vi "Fetch Multiple Records.vi"(0 "device session in":refnum<class "Device Session.lvclass">, 1 "starting record":u64, 2 "number of records":u64=1, 5 "fetch relative to":T1=enum."First Pretrigger Sample", 7 "number of samples":u64=1000, 9 "timeout (ms)":i32=1000, 11 "error in":errorcluster, 12 "fetch offset":i64, 13 "channel":u8=1) -> (4 "device session out":refnum<class "Device Session.lvclass">, 6 "data":dbl[][](array[numeric]), 8 "relativeX (samples)":dbl[](array[numeric]), 14 "requested records info":T2[](array[typedef]), 15 "error out":errorcluster)   [LabVIEW 2021, in "Device Session.lvclass"]
doc: "Fetches data from multiple records in an acquisition. No data is returned if this VI times out. You must run the <B>Initiate</B> VI before running this VI.\n\n<B>Input Parameters</B>\n\n<B>device session in</B> is a reference to the Device Session object, which contains a session to each instrument design library used in this sample project. This parameter is obtained from the 'Open Session' VI.\n\n<B>number of records</B> specifies the number of records to fetch samples from. The default value is 1.\n\n<B>starting record</B> specifies the record to retrieve. Index of the record numbers starts at 0.\n\n<B>fetch relative to</B> specifies the relative location within the acquired record from where the VI begins to fetch data.\n\n'First Sample': the fetch starts at the first sample acquired by the device. If the device wraps data in its memory buffer, the first sample is no longer available. In this case, the VI returns an error if 'fetch offset' specifies a location that is within the overwritten portion of the memory buffer.\n'Reference Trigger Sample': the fetch starts relative to the Reference Trigger.\n'First Pretrigger Sample': the fetch starts relative to the first pretrigger sample acquired. If you do not configure a Reference Trigger, 'First Pretrigger Sample' behaves the same as 'First Sample' because there are no pretrigger samples.\n'Most Recent Sample': the fetch starts relative to the most recently acquired sample. The value of 'fetch offset' must be negative. This VI doesn't support this option. Consider using the 'Fetch Single Record' VI instead.\n'Current Read Position': the fetch starts after the last fetched sample. This VI doesn't support this option. Consider using the 'Fetch Single Record' VI instead.\n\n<B>number of samples</B> specifies the number of samples to fetch. The default value is 1000.\n\n<B>timeout (ms)</B> specifies the time, in milliseconds, allotted for the Fetch Multiple Records VI to complete execution of each record before returning a timeout error. A value of -1 specifies that the VI waits until all data is available. A value of 0 is not supported. The default value is 10,000. You cannot abort a pending fetch using the Abort VI or Close VI.\n\n<B>fetch offset</B> specifies the offset relative to the position, which is specified by the 'fetch relative to' parameter, from which to start fetching data. Offset can be a positive or negative value. The default value is 0.\n\n<B>error in</B> describes error conditions that occur before this node runs. This input provides standard 'error in' functionality.\n\n<B>Output Parameters</B>\n\n<B>device session out</B> passes a reference to the session to the next VI.\n\n<B>data</B> returns the acquired records. Each waveform corresponds to a record. If the fetch contains multiple channels, all waveforms for a record are returned before proceeding to the next record. For example, a two-channel, two-record acquisition returns four waveforms:\narray index 0 = Channel0 Record0\narray index 1 = Channel1 Record0\narray index 2 = Channel0 Record1\narray index 3 = Channel1 Record1\n\n<B>relativeX (samples)</B> returns the relative positions from the trigger to the first sample in the acquired data.\n\n<B>requested records info</B> returns additional information about each record returned by 'data'. There is one element in the 'requested records info' array for each record.\n\n<B>requested records info.number of samples</B> returns the number of samples in the record.\n\n<B>requested records info.starting sample number</B> returns the sample number of the first sample in the returned record data. Sample numbers are zero-based. Sample numbers start at zero for each record and increment by one for each acquired sample.\n\n<B>requested records info.number of channels</B> returns the number of channels in the record data.\n\n<B>requested records info.timestamps</B> returns the timestamp values that were captured for the record.\n\n<B>error out</B> contains error information. This output provides standard 'error out' functionality."
uses:
  Device Session.lvclass
  <instrlib>/_niInstr/Multirecord Acquisition/Interface/v1/Host/Public/Requested Record Info.ctl
  <instrlib>/_niInstr/Multirecord Acquisition/Interface/v1/Host/Public/Fetch Relative To Enum.ctl
  Device Session.lvclass/Device Session.ctl
  <instrlib>/_niInstr/Multirecord Acquisition/Interface/v1/Host/Private/Fetch Multiple Records DBL Wrapper.vi
  <instrlib>/HSAI-RIO/Config/Group A/v1/Host/Main/niHSAI Group A Config v1 Host.lvclass
  <instrlib>/_niInstr/Multirecord Acquisition/Interface/v1/Host/niInstr Multirecord Acquisition v1 Host.lvclass
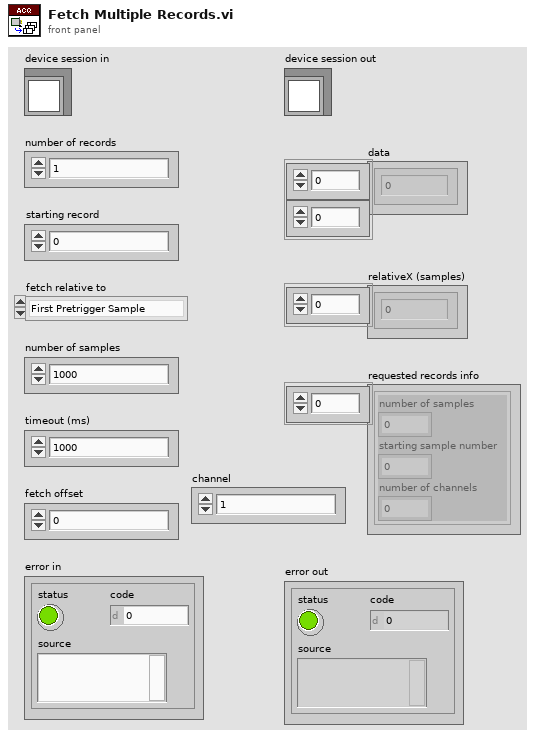
[diagram p1: front panel]
types:
  T1 = typedef "niInstr Multirecord Acquisition v1 Host.lvclass/Fetch Relative To Enum.ctl" = enum16{"First Sample", "Reference Trigger Sample", "First Pretrigger Sample", "Most Recent Sample", "Current Read Position"}
  T2 = typedef "niInstr Multirecord Acquisition v1 Host.lvclass/Requested Record Info.ctl" = cluster{"number of samples":u64, "starting sample number":u64, "number of channels":u64, "timestamps":u64[]}
  T3 = typedef "Device Session.lvclass/Device Session Object.ctl" = cluster{"fpga reference":T4, "reg bus":refnum<class "niInstr FIFO Register Bus v1 Host.lvclass">, "subsystem map":refnum<class "niInstr Subsystem Map v1 Host.lvclass">, "cal data":refnum<class "niHSAI Cal Data v1 Host.lvclass">, "config":refnum<class "niHSAI Group A Config v1 Host.lvclass">, "acquisition refs":refnum<class "niInstr Multirecord Acquisition v1 Host.lvclass">[], "acquisition 1":refnum<class "niInstr Multirecord Acquisition v1 Host.lvclass">, "number of selected acq channels":u8, "selected acq channels":bool[], "number of channels":u32, "configured channels":bool[], "acq configuration":cluster{"number of samples":u64, "number of records":u64, "pretrigger samples":u64}, "actual channel configuration":T5[], "sample clock rate (Hz)":dbl, "scaling coefficients":T9[]}
  T4 = typedef "Device Session.lvclass/FPGA Refnum.ctl" = refnum<k20>
  T5 = typedef "niHSAI Types v1 Host.lvlib/Channel Configuration.ctl" = cluster{"channel":u32, "coupling":T6, "impedance":T7, "bandwidth":T8, "vertical range":dbl, "vertical offset":dbl}
  T6 = typedef "niHSAI Types v1 Host.lvlib/Coupling.ctl" = enum8{"Default", "DC", "AC"}
  T7 = typedef "niHSAI Types v1 Host.lvlib/Impedance.ctl" = enum8{"Default", "1 mega ohm", "50 ohm"}
  T8 = typedef "niHSAI Types v1 Host.lvlib/Bandwidth.ctl" = enum8{"Default", "Full Bandwidth", "Anti-alias Filter", "150 MHz"}
  T9 = typedef "niInstr Multirecord Acquisition v1 Host.lvclass/Scaling Coefficient.ctl" = cluster{"gain":dbl, "offset":dbl}
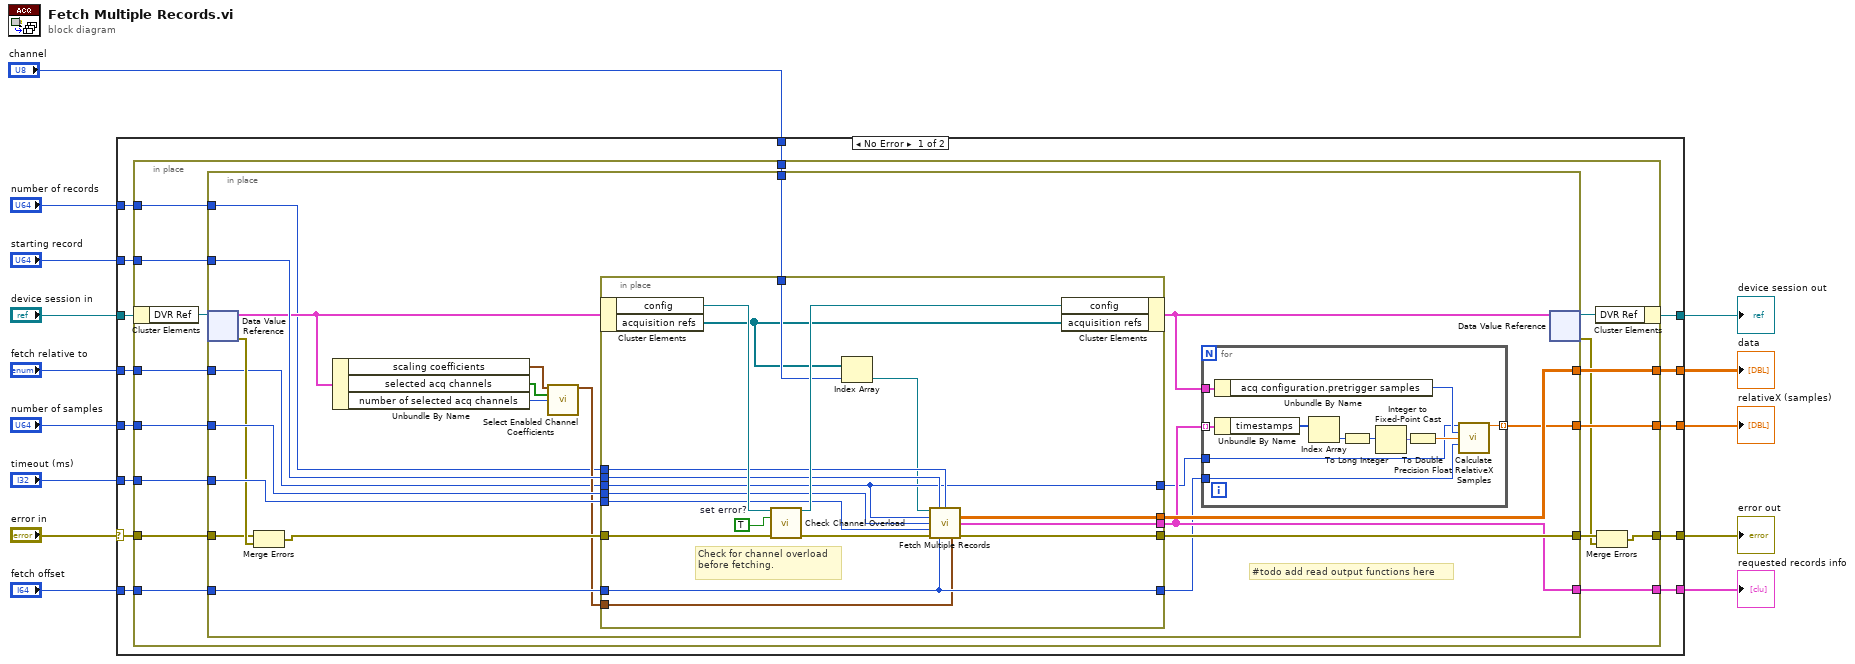
[diagram p0: block diagram]
diagram:
  n1 = case shown="No Error" "error in" {
    selector: "error in" -> [w28 w97]
    tunnel: [w23 w97] -> w2
    tunnel: "device session in" -> [w18 w96]
    tunnel: [w17 w96] -> w6
    tunnel: "number of samples" -> [w27 _]
    tunnel: "timeout (ms)" -> [w26 _]
    tunnel: "fetch offset" -> [w25 _]
    tunnel: "starting record" -> [w24 _]
    tunnel: "fetch relative to" -> [w22 _]
    tunnel: [w21 _] -> w5
    tunnel: [w20 _] -> w3
    tunnel: [w19 _] -> w4
    tunnel: "number of records" -> [w16 _]
    tunnel: "channel" -> [w15 _]
    frame No Error {
      n2 = in-place {
        in-place-border: w28 -> [w44]
        in-place-border: w27 -> [w43]
        in-place-border: w26 -> [w42]
        in-place-border: w25 -> [w41]
        in-place-border: w24 -> [w40]
        in-place-border: [w39] -> w23
        in-place-border: w22 -> [w37]
        in-place-border: [w36] -> w21
        in-place-border: [w35] -> w20
        in-place-border: [w34] -> w19
        in-place-border: w16 -> [w30]
        in-place-border: w15 -> [w29]
        n3 = in-place-cluster #1(w18) -> ("DVR Ref"=w32:refnum<data-value>)
        n4 = in-place {
          in-place-border: w44 -> [w62]
          in-place-border: [w66] -> w38
          in-place-border: w43 -> [w65]
          in-place-border: w42 -> [w64]
          in-place-border: w41 -> [w54]
          in-place-border: w40 -> [w59]
          in-place-border: w37 -> [w51]
          in-place-border: [w58] -> w36
          in-place-border: [w57] -> w35
          in-place-border: [w50] -> w34
          in-place-border: w30 -> [w48]
          in-place-border: w29 -> [w45]
          # "#todo add read output functions here"
          n5 = in-place-dvr #2(w32) -> (w52:T3, w63:errorcluster)
          n6 = Merge Errors(w62, w63) -> (w55:errorcluster)
          n7 = Unbundle By Name(w52) -> ("scaling coefficients"=w56:T9[], "selected acq channels"=w61:bool[], "number of selected acq channels"=w60:u8)
          n8 = call "Select Enabled Channel Coefficients.vi"("configured scaling coefficients"=w56, "selected acq channels to store"=w61, "number of selected acq channels to store"=w60) -> ("stored scaling coefficients"=w53:T9[])  [unwired: 12 in]
          n9 = in-place {
            in-place-border: [w88] -> w66
            in-place-border: w65 -> [w82]
            in-place-border: w64 -> [w81]
            in-place-border: w59 -> [w87]
            in-place-border: [w93] -> w58
            in-place-border: [w92] -> w50
            in-place-border: w55 -> [w91]
            in-place-border: w51 -> [w85]
            in-place-border: w54 -> [w84]
            in-place-border: w53 -> [w83]
            in-place-border: [w85] -> w47
            in-place-border: [w84] -> w46
            in-place-border: w48 -> [w86]
            in-place-border: w45 -> [w79]
            w94 = TRUE  # set error?
            # "Check for channel overload before fetching."
            n10 = in-place-cluster #3(w52) -> ("config"=w90:refnum<class "niHSAI Group A Config v1 Host.lvclass">, "acquisition refs"=w78:refnum<class "niInstr Multirecord Acquisition v1 Host.lvclass">[])
            n11 = call-dynamic "Check Channel Overload.vi"("session in"=w90, "set error? (T)"=w94, "error in"=w91) -> ("session out"=w89:refnum<class "niHSAI Group A Config v1 Host.lvclass">, "error out"=w95:errorcluster)  [unwired: 10 in, 1 out]
            n12 = Index Array(array=w78, index=w79) -> (element=w80:refnum<class "niInstr Multirecord Acquisition v1 Host.lvclass">)
            n13 = call-poly <instrlib>:"Fetch Multiple Records.vi"("session in"=w80, "starting record"=w87, "number of records"=w86, "fetch relative to"=w85, "number of samples"=w82, "timeout (ms)"=w81, "error in"=w95, "fetch offset"=w84, "scaling coefficients"=w83) -> ("data"=w93:dbl[][], "requested records info"=w92:T2[], "error out"=w88:errorcluster)  [unwired: 3 in, 1 out]
            n14 = in-place-cluster #3("config"=w89, "acquisition refs"=w78) -> (w49:T3)
          }
          n15 = for {
            tunnel: [w77] -> w57 mode=indexing
            tunnel: w50 -> [w72] mode=indexing
            tunnel: w49 -> [w70]
            tunnel: w47 -> [w68]
            tunnel: w46 -> [w67]
            n16 = Unbundle By Name(w70) -> ("acq configuration.pretrigger samples"=w69:u64)
            n17 = Unbundle By Name(w72) -> ("timestamps"=w74:u64[])
            n18 = Index Array(array=w74) -> (element=w73:u64)  [unwired: 1 in]
            n19 = To Long Integer(number=w73) -> (32bit integer=w75:i32)
            n20 = Integer to Fixed-Point Cast(integer=w75) -> (fixed-point=w76:fxp<+/-,32,5>)  [unwired: 1 in]
            n21 = To Double Precision Float(number=w76) -> (double precision float=w71:dbl)
            n22 = call "Calculate RelativeX Samples.vi"("fetch relative to"=w68, "pretrigger samples"=w69, "timestamps"=w71, "fetch offset"=w67) -> ("relativeX (samples)"=w77:dbl)  [unwired: 11 in]
          }
          n23 = in-place-dvr #2(w49) -> (w31:refnum<data-value>, w33:errorcluster)
        }
        n24 = in-place-cluster #1("DVR Ref"=w31) -> (w17:refnum<class "Device Session.lvclass">)
        n25 = Merge Errors(w38, w33) -> (w39:errorcluster)
      }
    }
    frame Error {
    }
  }
  "error out" <- w2
  "device session out" <- w6
  "requested records info" <- w4
  "data" <- w5
  "relativeX (samples)" <- w3
